vi "OF (SubVI).vi"() -> (0 "error out":errorcluster, 2 "Cluster":T2, 3 "Refnum out":T1)   [LabVIEW 2014]
uses:
  <vilib>/vision/Image Controls.llb/IMAQ Image.ctl
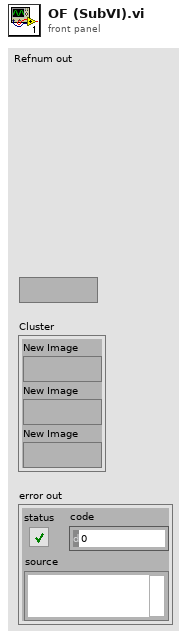
[diagram p1: front panel]
types:
  T1 = typedef "IMAQ Image.ctl" = refnum<image>
  T2 = cluster{"New Image":T1, "New Image":T1, "New Image":T1}
  T3 = typedef "Image Type" = u32
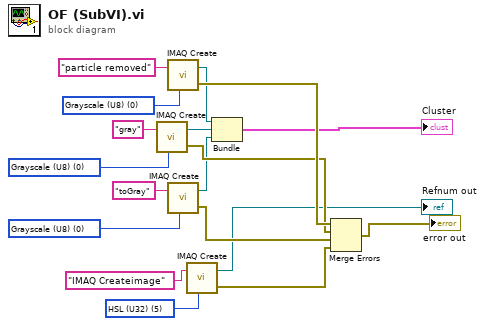
[diagram p0: block diagram]
diagram:
  w8 = T3 0 items=["Grayscale (U8)", "Grayscale (I16)", "Grayscale (SGL)", "Complex (CSG)", "RGB (U32)", "HSL (U32)", "RGB (U64)", "Grayscale (U16)"] ("Image Type")
  w6 = T3 0 items=["Grayscale (U8)", "Grayscale (I16)", "Grayscale (SGL)", "Complex (CSG)", "RGB (U32)", "HSL (U32)", "RGB (U64)", "Grayscale (U16)"] ("Image Type")
  w4 = T3 0 items=["Grayscale (U8)", "Grayscale (I16)", "Grayscale (SGL)", "Complex (CSG)", "RGB (U32)", "HSL (U32)", "RGB (U64)", "Grayscale (U16)"] ("Image Type")
  w2 = T3 5 items=["Grayscale (U8)", "Grayscale (I16)", "Grayscale (SGL)", "Complex (CSG)", "RGB (U32)", "HSL (U32)", "RGB (U64)", "Grayscale (U16)"] ("Image Type")
  n1 = call "IMAQ Create"("Image Name"="gray", "Image Type"=w8) -> ("New Image"=w11:T1, "error out"=w17:errorcluster)  [unwired: 3 in]
  n2 = call "IMAQ Create"("Image Name"="particle removed", "Image Type"=w4) -> ("New Image"=w10:T1, "error out"=w18:errorcluster)  [unwired: 3 in]
  n3 = call "IMAQ Create"("Image Name"="toGray", "Image Type"=w6) -> ("New Image"=w12:T1, "error out"=w16:errorcluster)  [unwired: 3 in]
  n4 = call "IMAQ Create"("Image Name"="IMAQ Createimage", "Image Type"=w2) -> ("New Image"=→"Refnum out":T1, "error out"=w15:errorcluster)  [unwired: 3 in]
  n5 = Bundle("New Image"=w10, "New Image"=w11, "New Image"=w12) -> (→"Cluster":T2)  [unwired: 1 in]
  n6 = Merge Errors(w18, w17, w16, w15) -> (→"error out":errorcluster)
